vi "Anti Tip.vi"(8 "Gear 2":bool, 9 "Motor Left":dbl, 10 "Motor Right":dbl, 11 "Drive Reduction":dbl) -> (0 "Gear 2?":bool, 2 "Motor Left Output":dbl, 3 "Motor Right Output":dbl)   [LabVIEW 2017]
uses:
  Robot Global Data.vi
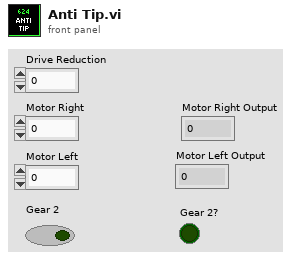
[diagram p1: front panel]
types:
  T1 = typedef "Dashboard Control Data.ctl" = cluster{"Drivetrain Settings Cluster":T2, "Intake Presets":T4, "Elevator Settings Cluster":T5, "Drivetrain Encoder Values":T7, "Auton Chooser":T8, "Auton Presets":cluster{"Start Position":dbl}, "Elevator Encoder Values":T9}
  T2 = typedef "Drivetrain Settings Cluster.ctl" = cluster{"Gyro Steer PID Gains":T3, "Distance Drive PID Gains":T3, "Drive Tolerance":dbl, "Gyro Tolerance":dbl, "Gyro Output":dbl, "Distance Output":dbl, "Y Power Multiplier":dbl, "Turn Power Multiplier":dbl, "Creep Rate":dbl, "Encoder Reset":bool, "DT Mode Modifier":enum16{"None, Default", "Cube", "Square"}, "Left Encoder Tick Constant":dbl, "Right Encoder Tick Constant":dbl, "Shift Speed":dbl, "Zero Gyro":bool}
  T3 = typedef "PID Gains Cluster.ctl" = cluster{"Integral Time":dbl, "Proportional Gain":dbl, "Derivative Time":dbl}
  T4 = typedef "Intake Presets.ctl" = cluster{"Idle Angle":dbl, "Mid Angle":dbl, "Low Angle":dbl, "Outtake Power":dbl, "Intake Power":dbl, "Unstuck":dbl, "Angle Tolerance":dbl, "Max Angle":dbl, "Max Current":dbl, "Current Trip Time":dbl, "Reset Encoder?":bool, "Encoder Scale":dbl, "PID gains":cluster{"proportional gain (Kc)":dbl, "integral time (Ti, min)":dbl, "derivative time (Td, min)":dbl}, "output range":cluster{"output high":dbl, "output low":dbl}, "IR Constant Pull Rate":dbl}
  T5 = typedef "Elevator Settings Cluster.ctl" = cluster{"Ground Height":dbl, "Switch Height":dbl, "Scale High Height ":dbl, "Scale Low Height":dbl, "Elevator PID Gains":T6, "Elevator Tolerance":dbl, "Reset Encoders":bool, "Encoder Scale":dbl, "Max Height":dbl, "Mid Height":dbl, "output range":cluster{"output high":dbl, "output low":dbl}, "Slow Down Tolerance":dbl, "Tick Constant":dbl, "Anti-tip Multiplier":dbl, "Slow Down Multiplier":dbl}
  T6 = typedef "PID Gains.ctl" = cluster{"proportional gain (Kc)":dbl, "integral time (Ti, min)":dbl, "derivative time (Td, min)":dbl}
  T7 = typedef "DT Encoder Values.ctl" = cluster{"Left Encoder":cluster{"Distance":dbl, "Speed":dbl, "Tick":dbl}, "Right Encoder":cluster{"Distance":dbl, "Speed":dbl, "Tick":dbl}}
  T8 = typedef "Auton Chooser.ctl" = cluster{"Left":bool, "Center":bool, "Right":bool, "Scale":bool, "Both":bool, "Switch":bool}
  T9 = typedef "Elevator Encoder Values.ctl" = cluster{"Encoder Values":cluster{"Distance":dbl, "Speed":dbl, "Tick":dbl}}
  T10 = typedef "Drivetrain Status Cluster.ctl" = cluster{"Throttle (Y)":dbl, "Steer (X)":dbl, "Drivetrain Mode":T11, "Brake?":bool, "Distance Drive Complete?":bool, "PID Drive Complete?":bool, "Creep Mode?":bool, "Gyro Steer Complete?":bool, "Gyro":dbl, "X Max Output":dbl, "X Min Output":dbl, "Y Max Output ":dbl, "Y Min Output":dbl, "Heading Target":dbl, "Distance Target":dbl, "2nd Gear":bool, "Drivetrain Encoder Values":T7}
  T11 = typedef "Drivetrain Mode.ctl" = enum16{"Manual", "Gyro Steer", "PID Drive", "Distance Drive", "Autonomous"}
  T12 = typedef "Elevator Status Cluster.ctl" = cluster{"Finished":bool, "Elevator Power":dbl, "Elevator State":T13, "Elevator Mode":T14, "Elevator Height":dbl, "At Bottom?":bool, "At Top?":bool, "Scale high?":bool, "PID Output":dbl}
  T13 = typedef "Elevator State.ctl" = enum16{"Idle", "Ground", "Mid", "Scale", "Switch"}
  T14 = typedef "Elevator Mode.ctl" = enum16{"Semi Auto", "Manual", "Auto"}
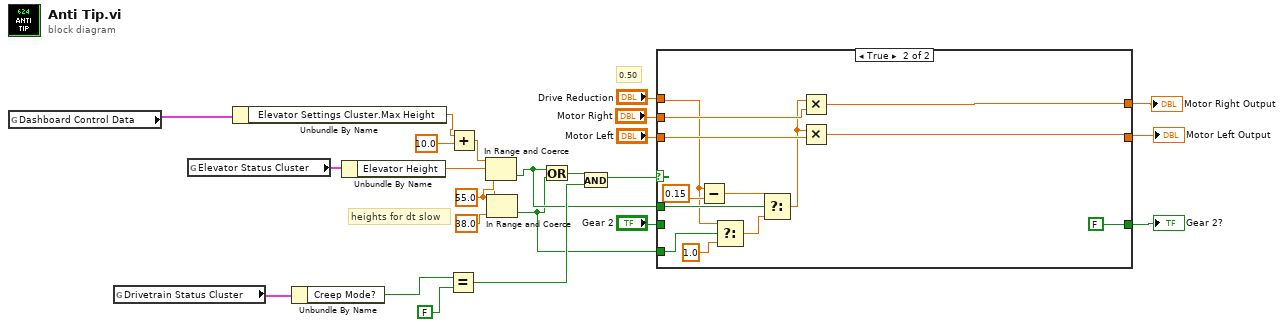
[diagram p0: block diagram]
diagram:
  w14 = 55.0 ("upper limit")
  # "heights for dt slow"
  # "0.50"
  n1 = global read "Robot Global Data.vi" "Dashboard Control Data"() -> (w13:T1)
  n2 = global read "Robot Global Data.vi" "Drivetrain Status Cluster"() -> (w11:T10)
  n3 = global read "Robot Global Data.vi" "Elevator Status Cluster"() -> (w23:T12)
  n4 = Unbundle By Name(w13) -> ("Elevator Settings Cluster.Max Height"=w3:dbl)
  n5 = Unbundle By Name(w11) -> ("Creep Mode?"=w9:bool)
  n6 = Unbundle By Name(w23) -> ("Elevator Height"=w4:dbl)
  n7 = Equal?(x=w9, y=FALSE) -> (x = y?=w8:bool)
  n8 = Add(x=w3, y=10.0) -> (x+y=w1:dbl)
  n9 = In Range and Coerce(upper limit=w1, x=w4, lower limit=w14) -> (In Range?=w6:bool)  [unwired: 1 out]
  n10 = In Range and Coerce(upper limit=w14, x=w4, lower limit=38.0) -> (In Range?=w5:bool)  [unwired: 1 out]
  n11 = Or(x=w6, y=w5) -> (x .or. y?=w12:bool)
  n12 = And(x=w12, y=w8) -> (x .and. y?=w7:bool)
  n13 = case shown="True" w7 {
    tunnel: [w26 w36] -> w22
    tunnel: "Motor Right" -> [w26 w39]
    tunnel: [w25 w37] -> w20
    tunnel: "Motor Left" -> [w25 w38]
    tunnel: "Gear 2" -> [w24 _]
    tunnel: [w24 FALSE] -> w17
    tunnel: "Drive Reduction" -> [_ w28]
    tunnel: w6 -> [_ w34]
    tunnel: w5 -> [_ w30]
    frame False {
    }
    frame True {
      n14 = Subtract(x=w28, y=0.15) -> (x-y=w33:dbl)
      n15 = Select(t=w28, s=w30, f=1.0) -> (s? t:f=w31:dbl)
      n16 = Select(t=w33, s=w34, f=w31) -> (s? t:f=w27:dbl)
      n17 = Multiply(x=w27, y=w39) -> (x*y=w36:dbl)
      n18 = Multiply(x=w27, y=w38) -> (x*y=w37:dbl)
    }
  }
  "Motor Right Output" <- w22
  "Motor Left Output" <- w20
  "Gear 2?" <- w17
